vi "Log Report.vi"(8 "error in (no error)":errorcluster, 9 "UUT.lvclass":refnum<class "UUT.lvclass">, 10 "Report in":refnum<class "Report.lvclass">, 11 "Sequence Engine in":refnum<class "Sequence Engine.lvclass">) -> (0 "error out":errorcluster, 2 "Report out":refnum<class "Report.lvclass">, 3 "Sequence Engine out":refnum<class "Sequence Engine.lvclass">)   [LabVIEW 2021, in "Sequence Engine.lvlib" / "Sequence Engine.lvclass"]
uses:
  Sequence Engine.lvclass
  PPLs/Report.lvlibp/Classes/Report/Report.lvclass
  UUT/UUT.lvclass
  PPLs/Report.lvlibp/Classes/Report/Report Metadata.ctl
  Sequence Engine.lvclass/Sequence Engine.ctl
  UUT/UUT.lvclass/UUT.ctl
  Test Result/Test Status.ctl
  Results Manager/Results Manager.lvclass
  Test Result/Test Result.lvclass
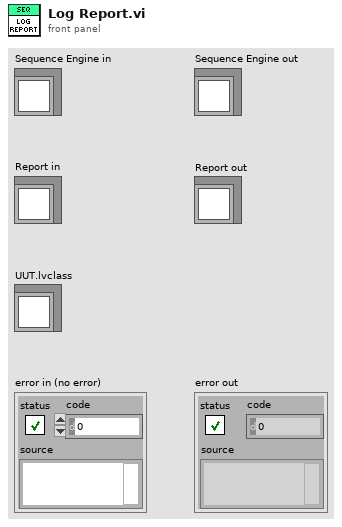
[diagram p1: front panel]
types:
  T1 = typedef "Report.lvlibp/Report.lvclass/Report Metadata.ctl" = cluster{"Model":string, "Serial Number":string, "Recipe Name":string, "Recipe Version":u16, "Username":string, "Test Status":string, "First Fail Test":string, "Start Time":timestamp, "Stop Time":timestamp, "Cycle Time (sec)":u16, "Execution Type":string}
  T2 = typedef "Sequence Engine.lvlib/Test Result.lvclass/Test Status.ctl" = enum16{"Pass", "Fail", "Aborted", "Skipped"}
  T3 = typedef "Sequence Engine.lvlib/Test Result.lvclass/Result Data.ctl" = cluster{"Test ID":u32, "Test Name":string, "Sub Test Name":string, "Test Status":T2, "Start Time":timestamp, "End Time":timestamp, "Duration (s)":dbl, "Expected Values":string, "Measured Values":string, "Remarks":string}
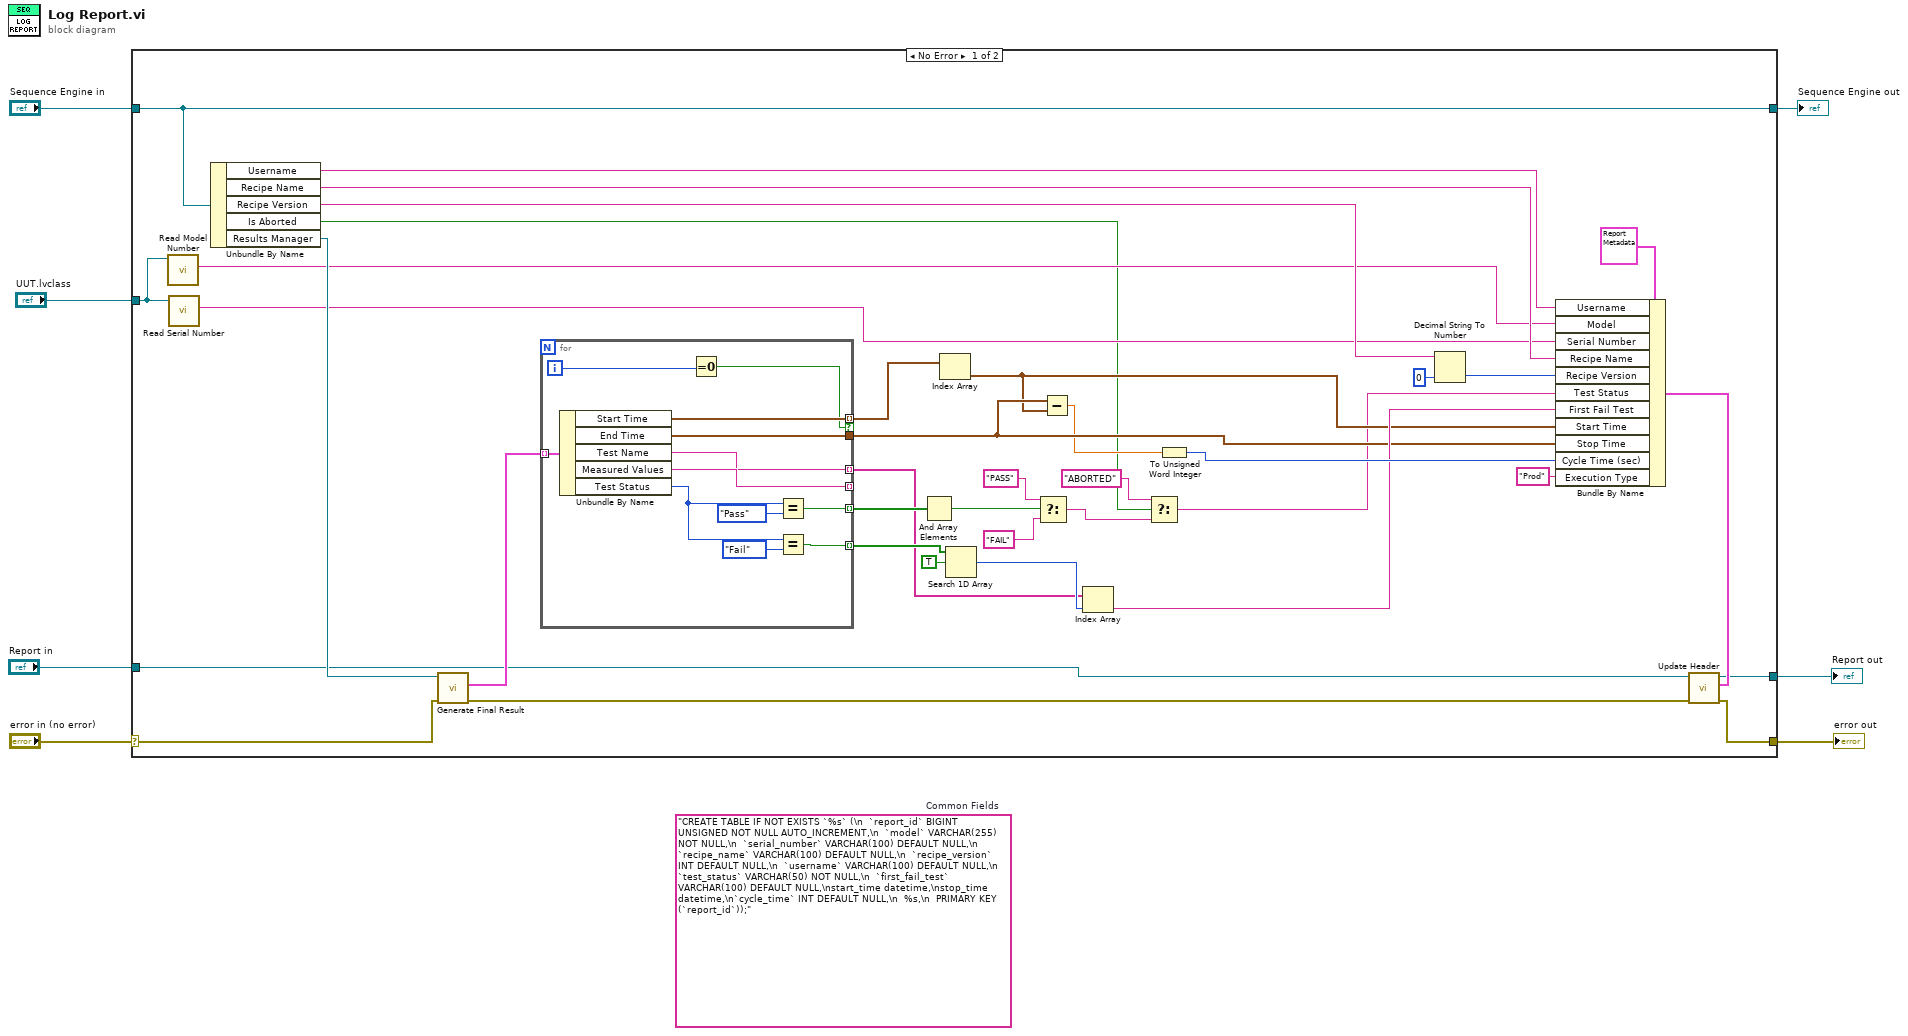
[diagram p0: block diagram]
diagram:
  (unwired) "CREATE TABLE IF NOT EXISTS `%s` (\n  `report_id` BIGINT UNSIGNED NOT NULL AUTO_INCREMENT,\n  `model` VARCHAR(255) NOT NULL,\n  `serial_number` VARCHAR(100) DEFAULT NULL,\n  `recipe_name` VARCHAR(100) DEFAULT NULL,\n  `recipe_version` INT DEFAULT NULL,\n  `username` VARCHAR(100) DEFAULT NULL,\n  `test_status` VARCHAR(50) NOT NULL,\n  `first_fail_test` VARCHAR(100) DEFAULT NULL,\nstart_time datetime,\nstop_time datetime,\n`cycle_time` INT DEFAULT NULL,\n  %s,\n  PRIMARY KEY (`report_id`));"  # Common Fields
  n1 = case shown="No Error" "error in (no error)" {
    selector: "error in (no error)" -> [w43 w59]
    tunnel: [w40 w59] -> w6
    tunnel: [w44 w58] -> w4
    tunnel: "Sequence Engine in" -> [w44 w58]
    tunnel: "Report in" -> [w18 w57]
    tunnel: [w17 w57] -> w2
    tunnel: "UUT.lvclass" -> [w15 _]
    frame No Error {
      n2 = call "Read Model Number.vi"("UUT in"=w15) -> ("Model Number"=w14:string)  [unwired: 8 in, 2 out]
      n3 = call "Read Serial Number.vi"("UUT in"=w15) -> ("Serial Number"=w16:string)  [unwired: 8 in, 2 out]
      n4 = Unbundle By Name(w44) -> ("Username"=w12:string, "Recipe Name"=w23:string, "Recipe Version"=w22:string, "Is Aborted"=w10:bool, "Results Manager"=w35:refnum<class "Results Manager.lvclass">)
      n5 = call-dynamic "Generate Final Result.vi"("error in (no error)"=w43, "Results Manager in"=w35) -> ("error out"=w42:errorcluster, "Array"=w41:T3[])  [unwired: 7 in, 1 out]
      n6 = for {
        tunnel: w41 -> [w56] mode=indexing
        tunnel: [w54] -> w33 mode=indexing
        tunnel: [w53] -> _ mode=indexing
        tunnel: [w50] -> w29 mode=indexing
        tunnel: [w49] -> w28 mode=indexing
        tunnel: [w48] -> w27 mode=indexing if=w46
        tunnel: [w45] -> w26
        i -> [w47]
        n7 = Unbundle By Name(w56) -> ("Start Time"=w48:timestamp, "End Time"=w45:timestamp, "Test Name"=w49:string, "Measured Values"=w53:string, "Test Status"=w51:T2)
        n8 = Equal To 0?(x=w47) -> (x = 0?=w46:bool)
        n9 = Equal?(x=w51, y=Test_Status."Pass") -> (x = y?=w54:bool)
        n10 = Equal?(x=w51, y=Test_Status."Fail") -> (x = y?=w50:bool)
      }
      n11 = And Array Elements(Boolean array=w33) -> (logical AND=w13:bool)
      n12 = Index Array(array=w27) -> (element=w25:timestamp)  [unwired: 1 in]
      n13 = Search 1D Array(1D array=w29, element=TRUE) -> (index of element=w31:i32)  [unwired: 1 in]
      n14 = Select(t="PASS", s=w13, f="FAIL") -> (s? t:f=w11:string)
      n15 = Subtract(x=w26, y=w25) -> (x-y=w24:dbl)
      n16 = Index Array(array=w28, index=w31) -> (element=w30:string)
      n17 = Select(t="ABORTED", s=w10, f=w11) -> (s? t:f=w8:string)
      n18 = To Unsigned Word Integer(number=w24) -> (unsigned 16bit integer=w36:u16)
      n19 = Decimal String To Number(string=w22, default (0L)=u16 0 ("default (0 I32)")) -> (number=w21:u16)  [unwired: 1 in, 1 out]
      n20 = Bundle By Name(cluster=T1 {"Model"="", "Serial Number"="", "Recipe Name"="", "Recipe Version"=0, "Username"="", "Test Status"="", "First Fail Test"="", "Start Time"=timestamp(0 s since 1904-01-01), "Stop Time"=timestamp(0 s since 1904-01-01), "Cycle Time (sec)"=0, "Execution Type"=""} ("Report Metadata"), "Username"=w12, "Model"=w14, "Serial Number"=w16, "Recipe Name"=w23, "Recipe Version"=w21, "Test Status"=w8, "First Fail Test"=w30, "Start Time"=w25, "Stop Time"=w26, "Cycle Time (sec)"=w36, "Execution Type"="Prod") -> (w34:T1)
      n21 = call "Update Header.vi"("error in (no error)"=w42, "Report Metadata"=w34, "Report in"=w18) -> ("error out"=w40:errorcluster, "Report out"=w17:refnum<class "Report.lvclass">)  [unwired: 7 in]
    }
    frame Error {
    }
  }
  "error out" <- w6
  "Sequence Engine out" <- w4
  "Report out" <- w2
